vi "SetPatterns.vi"(8 "Error In":errorcluster {"code" format="%.0x"}, 10 "Patterns":T1[](array[typedef]), 11 "Cards In":cluster{"Session":u32, "Card number":u32}[](array[cluster])) -> (0 "Error Out":errorcluster, 3 "Cards Out":cluster{"Session":u32, "Card number":u32}[](array[cluster]))   [LabVIEW 2012, in "Virtual-PGA.lvlib"]
doc: "This VI sets a pattern in the hardware. The relays are closed on the board based on the selected pattern."
uses:
  Virtual-PGA.lvlib
  Controls/Pattern.ctl
  Controls/Input.ctl
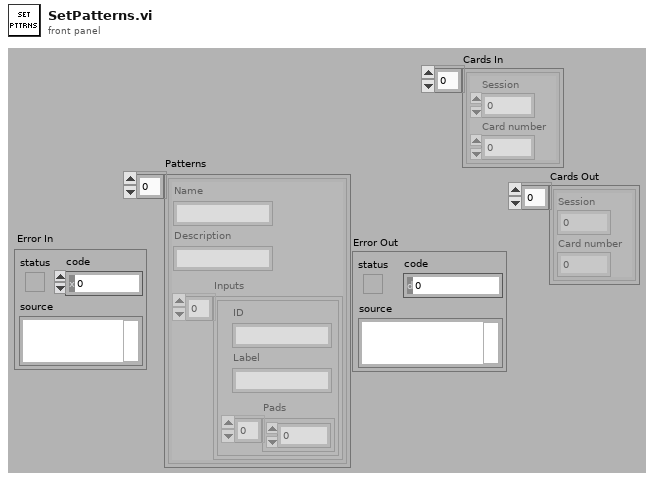
[diagram p1: front panel]
types:
  T1 = typedef "Virtual-PGA.lvlib/Pattern.ctl" = cluster{"Name":string, "Description":string, "Inputs":T2[]}
  T2 = typedef "Virtual-PGA.lvlib/Input.ctl" = cluster{"ID":string, "Label":string, "Pads":u32[]}
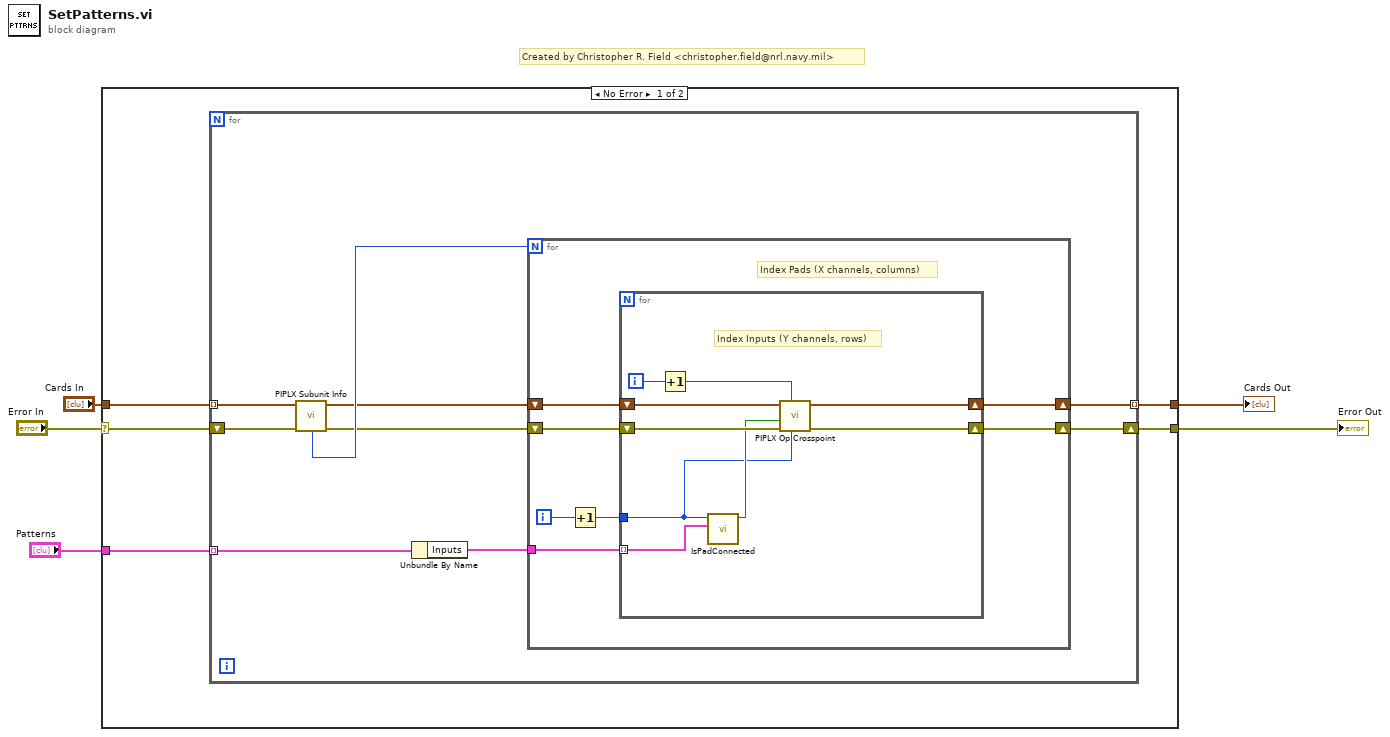
[diagram p0: block diagram]
diagram:
  # "Created by Christopher R. Field <christopher.field@nrl.navy.mil>"
  n1 = case shown="No Error" "Error In" {
    selector: "Error In" -> [w9 w37]
    tunnel: "Cards In" -> [w8 w36]
    tunnel: [w10 w37] -> w4
    tunnel: "Patterns" -> [w6 _]
    tunnel: [w7 w36] -> w1
    frame No Error {
      n2 = for {
        tunnel: w8 -> [w16] mode=indexing
        tunnel: w6 -> [w15] mode=indexing
        shift-right: [w18] -> w10
        shift-left: w9 -> [w17]
        tunnel: [w14] -> w7 mode=indexing
        n3 = call <instrlib>:"PIPLX Subunit Info.vi"("error in"=w17, "Input Handle"=w16) -> ("error out"=w11:errorcluster, "Output Handle"=w12:cluster{"Session":u32, "Card number":u32}, "Columns"=w13:u32)  [unwired: 5 in, 2 out]
        n4 = Unbundle By Name(w15) -> ("Inputs"=w19:T2[])
        n5 = for {
          N: w13 -> [_]
          tunnel: w19 -> [w25]
          shift-right: [w21] -> w18
          shift-left: w11 -> [w26]
          shift-right: [w20] -> w14
          shift-left: w12 -> [w22]
          i -> [w24]
          # "Index Pads (X channels, columns)"
          n6 = Increment(x=w24) -> (x+1=w23:i32)
          n7 = for {
            tunnel: w25 -> [w27] mode=indexing
            tunnel: w23 -> [w30]
            shift-right: [w33] -> w21
            shift-left: w26 -> [w32]
            shift-right: [w28] -> w20
            shift-left: w22 -> [w29]
            i -> [w35]
            # "Index Inputs (Y channels, rows)"
            n8 = Increment(x=w35) -> (x+1=w34:i32)
            n9 = call "IsPadConnected.vi"("Input"=w27, "Pad Number"=w30) -> ("Connected?"=w31:bool)  [unwired: 9 in]
            n10 = call <instrlib>:"PIPLX Op Crosspoint.vi"("Column"=w30, "Row"=w34, "error in"=w32, "Action"=w31, "Input Handle"=w29) -> ("error out"=w33:errorcluster, "Output Handle"=w28:cluster{"Session":u32, "Card number":u32})  [unwired: 5 in]
          }
        }
      }
    }
    frame Error {
    }
  }
  "Error Out" <- w4
  "Cards Out" <- w1
